vi "Connection.vi"(8 "error in (no error)":errorcluster, 11 "PLC_Module in":refnum<class "PLC_Module.lvclass">) -> (0 "error out":errorcluster, 2 "Connect_OK":bool, 3 "PLC_Module out":refnum<class "PLC_Module.lvclass">)   [LabVIEW 2025, in "PLC_Module.lvlib" / "PLC_Module.lvclass"]
uses:
  PLC_Module.lvclass
  PLC_Module.lvclass/PLC_Module.ctl
  PLC_Abstr/PLC_Abstr Messages/Connection Msg/Connection Msg.lvclass/Connection Msg.ctl
  <vilib>/ActorFramework/Message Enqueuer/Message Enqueuer.lvclass/Message Enqueuer.ctl
  Write Connect.vi
  Read ConnectConfig.vi
  <vilib>/ActorFramework/Message Enqueuer/Enqueue.vi
  PLC_Abstr/PLC_Abstr Messages/Connection Msg/Connection Msg.lvclass
  <vilib>/ActorFramework/Message Priority Queue/Priority Enqueue.vi
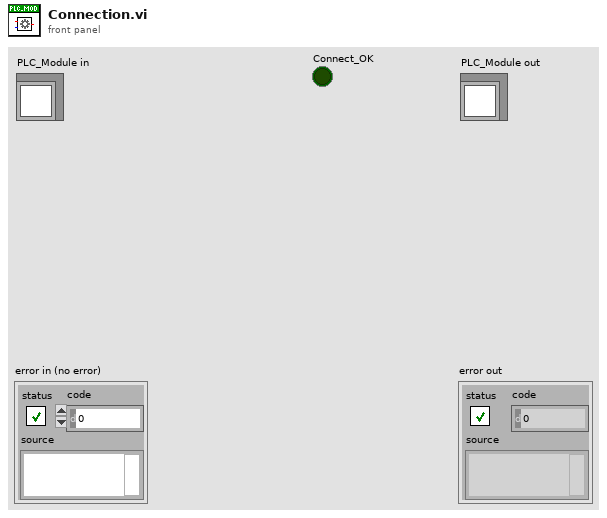
[diagram p1: front panel]
types:
  T1 = typedef "PLC_Module.lvlib/PLC_Module.lvclass/PLC_Connect_Config.ctl" = cluster{"IP Address":string, "Port":u16, "Timeout":i32}
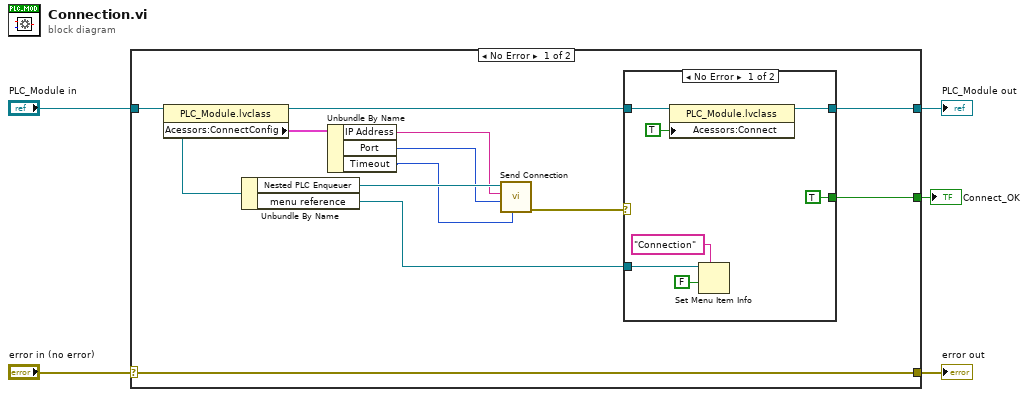
[diagram p0: block diagram]
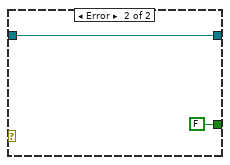
[diagram p2: hidden frame]
diagram:
  n1 = case shown="No Error" "error in (no error)" {
    selector: "error in (no error)" -> [w17 w28]
    tunnel: [w17 w28] -> w4
    tunnel: [w14 w27] -> w2
    tunnel: "PLC_Module in" -> [w16 w27]
    tunnel: [w6 _] -> w1
    frame No Error {
      n2 = property class="PLC_Module.lvclass"(reference=w16) -> (reference out=w11:refnum<class "PLC_Module.lvclass">, "Acessors:ConnectConfig"=w10:T1)  [unwired: 1 in, 1 out]
      n3 = Unbundle By Name(w16) -> ("Nested PLC Enqueuer"=w15:refnum<class "Message Enqueuer.lvclass">, "menu reference"=w12:refnum<k9>)
      n4 = Unbundle By Name(w10) -> ("IP Address"=w9:string, "Port"=w8:u16, "Timeout"=w7:i32)
      n5 = call "Send Connection.vi"("Timeout"=w7, "Port"=w8, "IP Address"=w9, "Message Enqueuer"=w15) -> ("error out"=w13:errorcluster)  [unwired: 6 in, 1 out]
      n6 = case shown="No Error" w13 {
        tunnel: w11 -> [w24 w26]
        tunnel: [w23 w26] -> w14
        tunnel: w12 -> [w19 _]
        tunnel: [TRUE FALSE] -> w6
        frame No Error {
          n7 = property class="PLC_Module.lvclass"(reference=w24, "Acessors:Connect"=TRUE ("Connect")) -> (reference out=w23:refnum<class "PLC_Module.lvclass">)  [unwired: 1 in, 1 out]
          n8 = Set Menu Item Info(7:"Connection" ("item tag"), 9:FALSE ("enabled"), 11:w19) -> ()  [unwired: 4 in, 2 out]
        }
        frame Error {
        }
      }
    }
    frame Error {
    }
  }
  "error out" <- w4
  "PLC_Module out" <- w2
  "Connect_OK" <- w1
